vi "Close.vi"(8 "Error In":errorcluster, 11 "AD2 I2C In":refnum<class "AD2 I2C.lvclass">=refnum) -> (0 "Error Out":errorcluster, 2 "WaveForms Session Out":T1, 3 "AD2 I2C Out":refnum<class "AD2 I2C.lvclass">)   [LabVIEW 2020, in "lv_i2c_ad2.lvlib" / "AD2 I2C.lvclass"]
uses:
  AD2 I2C.lvclass
  <vilib>/miidas/lv_i2c_ad2/WFT Session.ctl
  AD2 I2C.lvclass/AD2 I2C.ctl
  <vilib>/miidas/lv_i2c_ad2/lv_waveforms_toolkit.lvlib
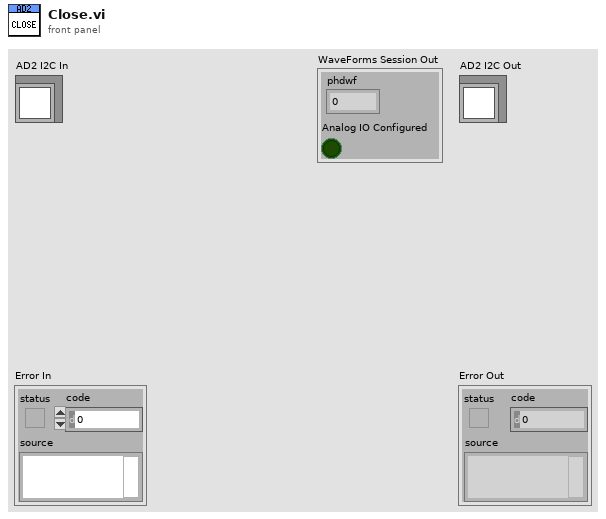
[diagram p1: front panel]
types:
  T1 = typedef "lv_waveforms_toolkit.lvlib/WFT Session.ctl" = cluster{"phdwf":i32, "Analog IO Configured":bool}
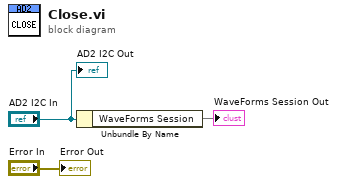
[diagram p0: block diagram]
diagram:
  n1 = Unbundle By Name("AD2 I2C In") -> ("WaveForms Session"=→"WaveForms Session Out")
  "Error Out" <- "Error In"
  "AD2 I2C Out" <- "AD2 I2C In"
